vi "VI Server_Get Cluster Controls Refferences With Merging.vi"(7 "Cluster Label":string, 8 "error in":errorcluster, 11 "VI Server Cluster":T1={"Labels"=["Label", "Size", "Font", "Heght", "Width", "Ledding Denominator", "Ledding Nominator", "Label Number", "Microstep Resolution", "X", "Y", "Z", "Italic?", "Underlined?"], "Refs"=[], "VI Ref"=refnum}) -> (0 "error out":errorcluster, 3 "VI Server Cluster.DUP":T1={"Labels"=["Label", "Size", "Font", "Heght", "Width", "Ledding Denominator", "Ledding Nominator", "Label Number", "Microstep Resolution", "X", "Y", "Z", "Italic?", "Underlined?"], "Refs"=[], "VI Ref"=refnum}, 4 "Claster.ControlLabels":string[](array[string]) caption="ClasterControlLabels", 6 "Claster.ControRefs":refnum<vi>[](array[refnum]) caption="ClasterControRefs")   [LabVIEW 2020, in "VI Server Toolkit LV2013.lvlib"]
doc: "Retrieves cluster's content labels and associated references and adds them to VI Server Cluster.\nThese controls can be accessed via VI Server Tools.\nPlease keep in mind the labels should be unique in order to be properly identified."
uses:
  VI Server Toolkit LV2013.lvlib
  VI Server_TypeDefs/VI Server_RefsCluster.ctl
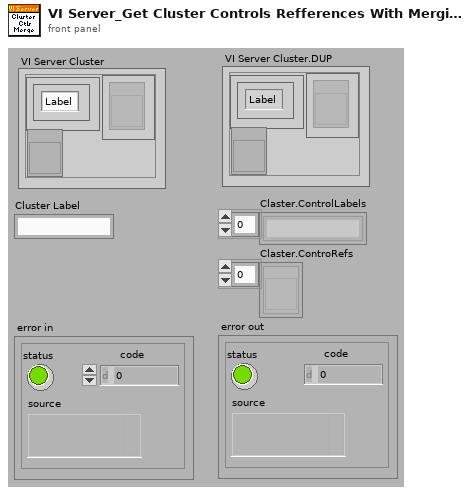
[diagram p1: front panel]
types:
  T1 = typedef "VI Server_RefsCluster.ctl" = cluster{"Labels":string[], "Refs":refnum<vi>[], "VI Ref":refnum<vi>}
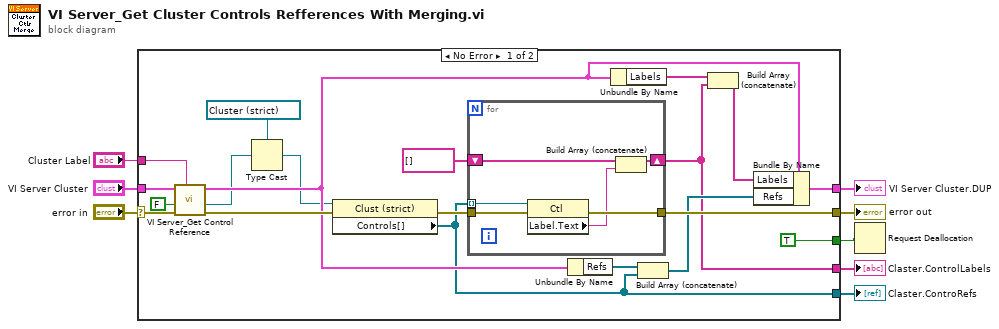
[diagram p0: block diagram]
diagram:
  n1 = case shown="No Error" "error in" {
    selector: "error in" -> [w20 w35]
    tunnel: "VI Server Cluster" -> [w18 _]
    tunnel: [w28 w35] -> w7
    tunnel: [w21 _] -> w5
    tunnel: "Cluster Label" -> [w16 _]
    tunnel: [w12 _] -> w2
    tunnel: [w11 _] -> w3
    tunnel: [TRUE _] -> w1
    frame No Error {
      n2 = call "VI Server_Get Control Reference.vi"("Label"=w16, "error in"=w20, "Single Instance (T)"=FALSE, "VI Server Cluster"=w18) -> ("error out"=w19:errorcluster, "Control Reference (Generic)"=w15:refnum<vi>, "VI Server Cluster.DUP"=w17:T1)  [unwired: 4 in, 1 out]
      n3 = Type Cast(type=refnum<vi> refnum ("VI ServerCluster 2"), x=w15) -> (*(type *) &x=w14:refnum<vi>)
      n4 = property class="Clust (strict)"(reference=w14, error in=w19) -> (error out=w27:errorcluster, "Controls[]"=w12:refnum<vi>[])  [unwired: 1 out]
      n5 = for {
        tunnel: w27 -> [w29]
        tunnel: [w34] -> w28
        tunnel: w12 -> [w30] mode=indexing
        shift-right: [w31] -> w11
        shift-left: string[] [] -> [w33]
        n6 = property class="Ctl"(reference=w30, error in=w29) -> (error out=w34:errorcluster, "Label.Text"=w32:string)  [unwired: 1 out]
        n7 = Build Array (concatenate)(w33, w32) -> (w31:string[])
      }
      n8 = Unbundle By Name(w17) -> ("Refs"=w24:refnum<vi>[])
      n9 = Unbundle By Name(w17) -> ("Labels"=w25:string[])
      n10 = Build Array (concatenate)(w24, w12) -> (w22:refnum<vi>[])
      n11 = Build Array (concatenate)(w25, w11) -> (w23:string[])
      n12 = Bundle By Name(cluster=w17, "Labels"=w23, "Refs"=w22) -> (w21:T1)
    }
    frame Error {
    }
  }
  "error out" <- w7
  "VI Server Cluster.DUP" <- w5
  "Claster.ControlLabels" <- w3
  "Claster.ControRefs" <- w2
  n13 = Request Deallocation(w1) -> ()
